vi "_CSMOFGV Get.vi"(8 "Error in":errorcluster caption="Error in (no error)", 10 "Message":string, 11 "Name(\"\" to use uuid) in":string) -> (0 "Error out":errorcluster, 3 "CSM-Obj":T1={"Requested Name"="", "Module Name"="", "Mode"=enum."Stand Alone", "Queue"=refnum, "CSM-Data"=refnum, "User Event"=refnum, "Status Change Event"=refnum, "Allowed Messages"=[], "Mode-Data"=refnum, "Group Name"="", "Exit Event"=refnum}, 4 "Name":string)   [LabVIEW 2020, in "Communicable State Machine.lvlib"]
uses:
  Communicable State Machine.lvlib
  _CSMObj.ctl
  Priority Queue.lvclass
  _CSM_MODE.ctl
  _CSMObj-Data.ctl
  _CSM Status Change Event Data.ctl
  _CSMObj-ModeData.ctl
  _CSMOFGVOPER.ctl
  global-CSMQ FGV Change Flag.vi
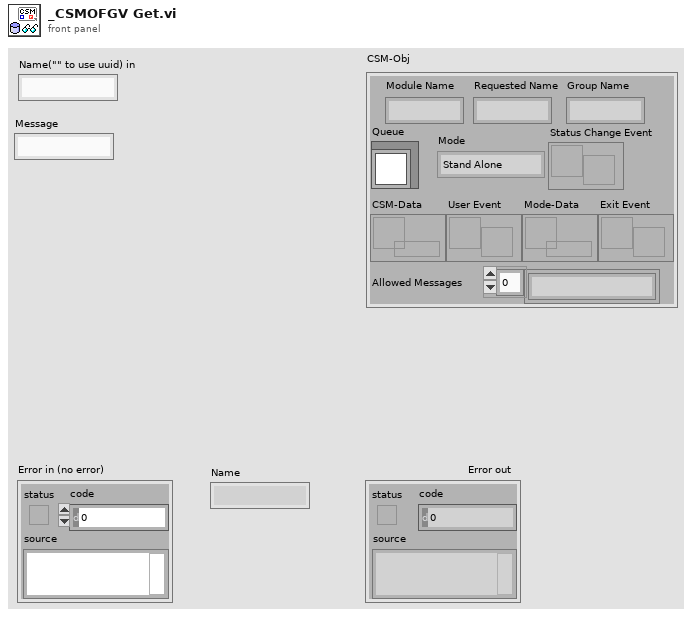
[diagram p1: front panel]
types:
  T1 = typedef "Communicable State Machine.lvlib/_CSMObj.ctl" = cluster{"Requested Name":string, "Module Name":string, "Mode":T2, "Queue":refnum<class "Priority Queue.lvclass">, "CSM-Data":refnum<data-value>, "User Event":refnum<user-event>, "Status Change Event":refnum<user-event>, "Allowed Messages":string[], "Mode-Data":refnum<data-value>, "Group Name":string, "Exit Event":refnum<user-event>}
  T2 = typedef "Communicable State Machine.lvlib/_CSM_MODE.ctl" = enum16{"Not Exist", "Stand Alone", "CSM", "Worker Agent", "Worker", "Chain", "Chain Node"}
  T3 = typedef "Communicable State Machine.lvlib/_CSMOFGVOPER.ctl" = enum16{"Create If not Exist", "Get By Name", "List", "Check If Name Exists", "Release", "Module Status", "Create Status Event Handler", "Destroy Status Event Handler"}
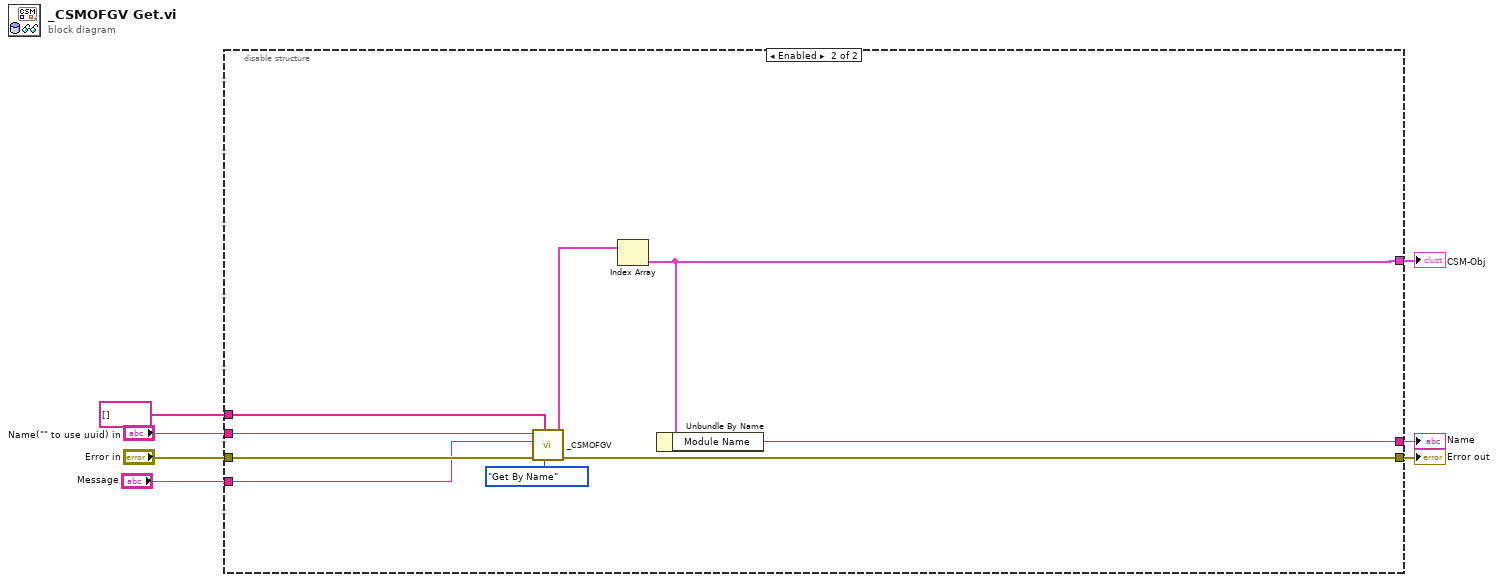
[diagram p0: block diagram]
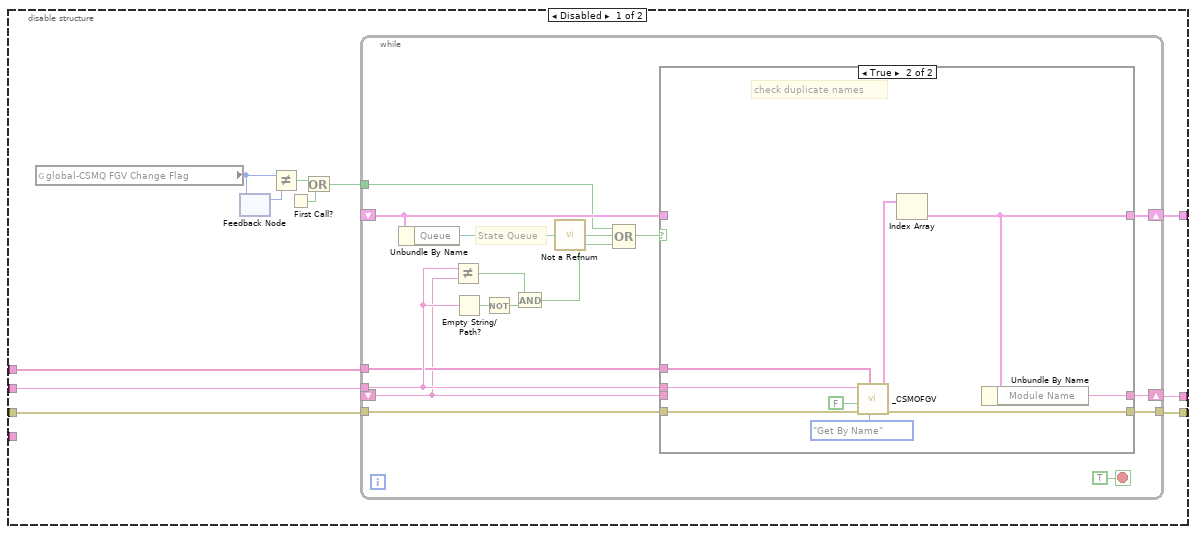
[diagram p2: hidden frame]
diagram:
  n1 = disable-structure shown="Enabled" {
    disable-tunnel: [w18 w50] -> w7
    disable-tunnel: "Error in" -> [w17 w52]
    disable-tunnel: [w16 w51] -> w5
    disable-tunnel: "Name(\"\" to use uuid) in" -> [w15 w54]
    disable-tunnel: [w14 w49] -> w3
    disable-tunnel: string[] [] ("Allowed Messages(Empty for all)") -> [w12 w53]
    disable-tunnel: "Message" -> [_ w48]
    frame Disabled {
      n2 = global read "global-CSMQ FGV Change Flag.vi" "global-CSMQ FGV Change Flag"() -> (w8:u64)
      n3 = feedback #1() -> (w9:u64)  [unwired: 1 in]
      n4 = feedback-in #1(w8) -> ()
      n5 = Not Equal?(x=w8, y=w9) -> (x != y?=w11:bool)
      n6 = First Call?() -> (First Call?: T/F=w10:bool)
      n7 = Or(x=w11, y=w10) -> (x .or. y?=w13:bool)
      n8 = while {
        shift-right: [w33] -> w18
        shift-left: _ -> [w19]
        shift-right: [w32] -> w14
        shift-left: _ -> [w26]
        tunnel: w17 -> [w31]
        tunnel: [w30] -> w16
        tunnel: w15 -> [w27]
        tunnel: w13 -> [w21]
        tunnel: w12 -> [w20]
        stop <- TRUE stop-if-true
        # "State Queue"
        n9 = Unbundle By Name(w26) -> ("Queue"=w25:refnum<class "Priority Queue.lvclass">)
        n10 = Not Equal?(x=w27, y=w19) -> (x != y?=w24:bool)
        n11 = Empty String/Path?(string/path=w27) -> (empty?=w23:bool)
        n12 = Not(x=w23) -> (.not. x?=w22:bool)
        n13 = And(x=w24, y=w22) -> (x .and. y?=w28:bool)
        n14 = call "Not a Refnum.vi"("Priority Queue.lvclass"=w25) -> ("NaN/Path/Refnum?"=w34:bool)  [unwired: 4 in]
        n15 = Compound Arithmetic op=OR(w21, w34, w28) -> (w29:bool)
        n16 = case shown="True" w29 {
          tunnel: w19 -> [w38 _]
          tunnel: [w38 w39] -> w33
          tunnel: [w37 w40] -> w32
          tunnel: w26 -> [w37 _]
          tunnel: w31 -> [w36 w43]
          tunnel: [w36 w45] -> w30
          tunnel: w27 -> [_ w44]
          tunnel: w20 -> [_ w42]
          frame False {
          }
          frame True {
            # "check duplicate names"
            n17 = call "_CSMOFGV.vi"("Operation"=_CSMOFGVOPER."Get By Name", "Allowed Messages(Empty for all)"=w42, "Error in"=w43, 9:FALSE ("create if not found? (T)"), "Name(\"\" to use uuid) in"=w44) -> ("Error out"=w45:errorcluster, "Array"=w47:T1[])  [unwired: 4 in, 1 out]
            n18 = Index Array(array=w47) -> (element=w40:T1)  [unwired: 1 in]
            n19 = Unbundle By Name(w40) -> ("Module Name"=w39:string)
          }
        }
      }
    }
    frame Enabled {
      n20 = call "_CSMOFGV.vi"("Operation"=_CSMOFGVOPER."Get By Name", "Allowed Messages(Empty for all)"=w53, "Error in"=w52, "Reference"=w48, "Name(\"\" to use uuid) in"=w54) -> ("Error out"=w51:errorcluster, "Array"=w56:T1[])  [unwired: 4 in, 1 out]
      n21 = Index Array(array=w56) -> (element=w49:T1)  [unwired: 1 in]
      n22 = Unbundle By Name(w49) -> ("Module Name"=w50:string)
    }
  }
  "Error out" <- w5
  "CSM-Obj" <- w3
  "Name" <- w7
